vi "writeToXML.vi"(8 "error in (no error)":errorcluster, 10 "Class Label":string, 11 "NewScienceTarget in":refnum<class "NewScienceTarget.lvclass">) -> (0 "error out":errorcluster, 2 "XML out":string, 3 "NewScienceTarget out":refnum<class "NewScienceTarget.lvclass">)   [LabVIEW 2022 SP3, in "TCSDataDefinitions.lvlib" / "TCSPublicStatus.lvlib" / "NewScienceTarget.lvclass"]
uses:
  NewScienceTarget.lvclass
  <userlib>/Common/UnitsAndXML/FlattenItemWithUnitToXML/FlattenLengthToXML/LengthUnit.ctl
  NewScienceTarget.lvclass/NewScienceTarget.ctl
  TCSCommand/TargetConfiguration/ScienceTargetConfiguration/ScienceTargetConfiguration.lvclass
  TCSCommand/TargetConfiguration/Target/FixedTarget/RADecParameters/RADecParameters.lvclass
  <userlib>/Common/UnitsAndXML/UnitsAndXML.lvlib
  <userlib>/Common/XML/XMLGenerator/XMLGenerator.lvclass
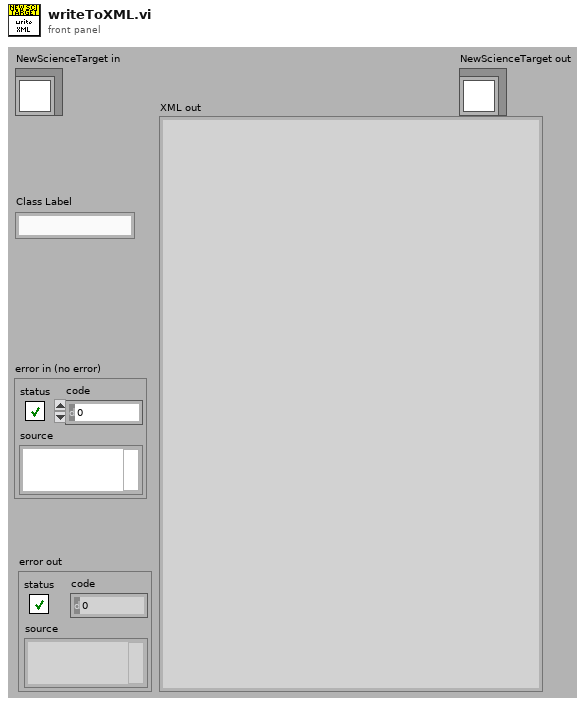
[diagram p1: front panel]
types:
  T1 = typedef "UnitsAndXML.lvlib/LengthUnit.ctl" = enum16{"m", "Angstrom", "AU", "chain", "cm", "cubit", "fathom", "fermi", "ft", "furlong", "hubble", "in", "ly", "mi", "mm", "rod", "um", "yd"}
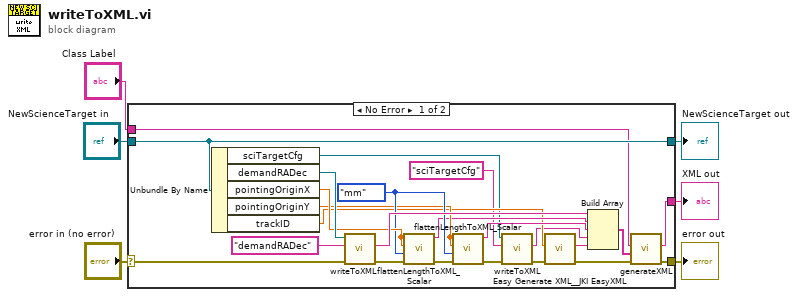
[diagram p0: block diagram]
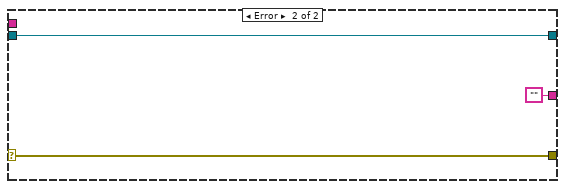
[diagram p2: hidden frame]
diagram:
  n1 = case shown="No Error" "error in (no error)" {
    selector: "error in (no error)" -> [w27 w33]
    tunnel: [w14 w33] -> w5
    tunnel: [w30 w32] -> w3
    tunnel: "NewScienceTarget in" -> [w30 w32]
    tunnel: "Class Label" -> [w16 _]
    tunnel: [w13 ""] -> w1
    frame No Error {
      w24 = LengthUnit."mm" ("lengthUnitInXML")
      n2 = Unbundle By Name(w30) -> ("sciTargetCfg"=w12:refnum<class "ScienceTargetConfiguration.lvclass">, "demandRADec"=w29:refnum<class "RADecParameters.lvclass">, "pointingOriginX"=w25:dbl[unit], "pointingOriginY"=w23:dbl[unit], "trackID"=w18:dbl)
      n3 = call-dynamic "writeToXML.vi"("error in (no error)"=w27, "Class Label"="demandRADec", "RADecParameters in"=w29) -> ("error out"=w21:errorcluster, "XML out"=w26:string)  [unwired: 6 in, 1 out]
      n4 = call <userlib>:"flattenLengthToXML_Scalar.vi"("error in (no error)"=w21, "lengthUnitInXML"=w24, "lengthAgain"=w25, "length"=w25) -> ("error out"=w22:errorcluster, "xmlString"=w20:string)  [unwired: 6 in]
      n5 = call <userlib>:"flattenLengthToXML_Scalar.vi"("error in (no error)"=w22, "lengthUnitInXML"=w24, "lengthAgain"=w23, "length"=w23) -> ("error out"=w10:errorcluster, "xmlString"=w19:string)  [unwired: 6 in]
      n6 = call-dynamic "writeToXML.vi"("error in (no error)"=w10, "ClassLabel"="sciTargetCfg" ("Class Label"), "ScienceTargetConfiguration in"=w12) -> ("error out"=w9:errorcluster, "XML out"=w7:string)  [unwired: 6 in, 1 out]
      n7 = call <vilib>:"Easy Generate XML__JKI EasyXML.vi"("error in (no error)"=w9, "LabVIEW Data"=w18) -> ("error out"=w15:errorcluster, "XML String"=w8:string)  [unwired: 8 in]
      n8 = Build Array(w26, w20, w19, w7, w8) -> (w17:string[])
      n9 = call <userlib>:"generateXML.vi"("error in"=w15, "childrenXML"=w17, "elementName"=w16) -> ("error out"=w14:errorcluster, "XML out"=w13:string)  [unwired: 6 in, 1 out]
    }
    frame Error {
    }
  }
  "error out" <- w5
  "NewScienceTarget out" <- w3
  "XML out" <- w1
